vi "gear.vi"() -> ()   [LabVIEW 2016, in "Shared resources RT.lvlib"]
uses:
  Shared resources RT.lvlib
panel:
  in  "Gear":enum16{"7", "6", "5", "4", "3", "2", "1"}(ring)=enum."4"
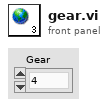
[diagram p1: front panel]
diagram:
